vi "setfIRF.vi"(8 "error in (no error)":errorcluster, 10 "fIRF":dbl[](array[numeric]), 11 "LaguerreDeconEngineClass in":refnum<class "LaguerreDeconEngineClass.lvclass">) -> (0 "error out":errorcluster, 3 "LaguerreDeconEngineClass out":refnum<class "LaguerreDeconEngineClass.lvclass">)   [LabVIEW 2024, in "LaguerreDeconEngineClass.lvclass"]
uses:
  LaguerreDeconEngineClass.lvclass
  LaguerreDeconEngineClass.lvclass/LaguerreDeconEngineClass.ctl
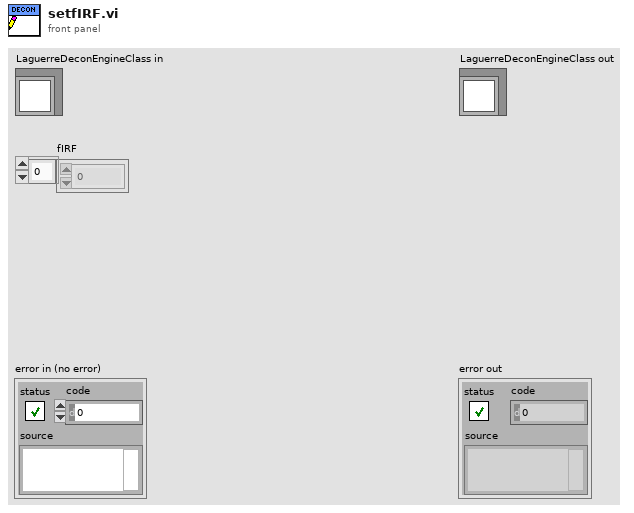
[diagram p1: front panel]
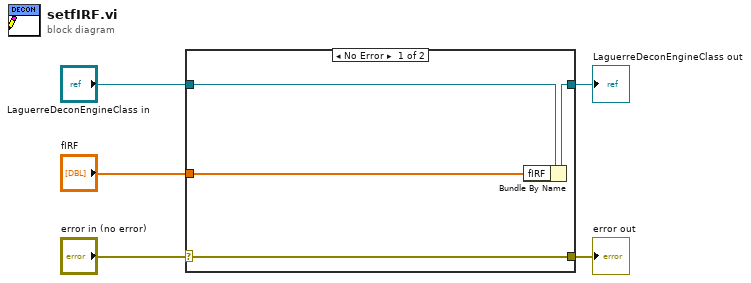
[diagram p0: block diagram]
diagram:
  n1 = case shown="No Error" "error in (no error)" {
    selector: "error in (no error)" -> [w9 w10]
    tunnel: [w9 w10] -> w4
    tunnel: [w7 w11] -> w2
    tunnel: "LaguerreDeconEngineClass in" -> [w8 w11]
    tunnel: "fIRF" -> [w6 _]
    frame No Error {
      n2 = Bundle By Name(cluster=w8, "fIRF"=w6) -> (w7:refnum<class "LaguerreDeconEngineClass.lvclass">)
    }
    frame Error {
    }
  }
  "error out" <- w4
  "LaguerreDeconEngineClass out" <- w2
